vi "Actor Receive Core.vi"(10 "Msg in":refnum<class "Msg Strategy.lvclass">, 11 "Destroying Self Actor State in":refnum<class "Destroying Self Actor State.lvclass">) -> (2 "Msg out":refnum<class "Msg Strategy.lvclass">)   [LabVIEW 2021, in "LVCAM.lvlib" / "Destroying Self Actor State.lvclass"]
uses:
  Destroying Self Actor State.lvclass
  Msg Strategy/Msg Strategy.lvclass
  Msgs/Actor Last Ack/Actor Last Ack Msg Strategy/Actor Last Ack Msg Strategy.lvclass
  C:/PPLs/LabVIEW-Composed-Actor-Model-LVCAM/LabVIEW-Composed-Actor-Model-LVCAM/LVCAM/LVCAM/Msg Strategy/Msg Strategy.lvclass
  Msgs/Actor Destroy/Actor Destroy Msg Strategy/Actor Destroy Msg Strategy.lvclass
  Destroying Self Actor State.lvclass/Destroying Self Actor State.ctl
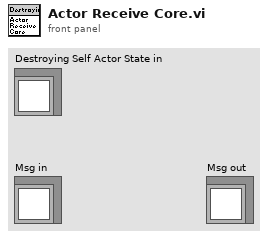
[diagram p1: front panel]
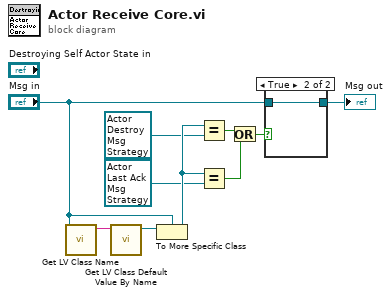
[diagram p0: block diagram]
diagram:
  n1 = call <vilib>:"Get LV Class Name.vi"("object"="Msg in") -> ("class name"=w10:string)  [unwired: 9 in, 1 out]
  n2 = call <vilib>:"Get LV Class Default Value By Name.vi"("class name"=w10) -> ("object"=w9:refnum<class>)  [unwired: 9 in, 1 out]
  n3 = To More Specific Class(target class="Msg in", reference=w9) -> (specific class reference=w7:refnum<class "Msg Strategy.lvclass">)  [unwired: 1 in, 1 out]
  n4 = Equal?(x=w7, y=refnum<class "Actor Destroy Msg Strategy.lvclass"> refnum ("LVCAM Destroy Self.lvlib:LVCAM Destroy Self Msg.lvclass")) -> (x = y?=w8:bool)
  n5 = Equal?(x=w7, y=refnum<class "Actor Last Ack Msg Strategy.lvclass"> refnum ("LVCAM Nest Destroyed.lvlib:LVCAM Nest Destroyed Msg.lvclass")) -> (x = y?=w5:bool)
  n6 = Or(x=w8, y=w5) -> (x .or. y?=w3:bool)
  n7 = case shown="True" w3 {
    tunnel: [_ w11] -> w1
    tunnel: "Msg in" -> [_ w11]
    frame False {
    }
    frame True {
    }
  }
  "Msg out" <- w1
